vi "IOC shared memory de-initialize.vi"(0 "shared memory in":T2, 3 "Shared memory cluster":T1) -> ()   [LabVIEW 2020, in "linuxSharedMemory.lvlib"]
uses:
  linuxSharedMemory.lvlib
  <vilib>/NI/NI Linux RT IPC/Shared Memory/Controls/reference.ctl
  <vilib>/NI/NI Linux RT IPC/Shared Memory/Classes/Shared Memory/Shared Memory.lvclass
  controls/sm_cluster.ctl
  <vilib>/NI/NI Linux RT IPC/Shared Memory/Linux RT IPC.Shared Memory.lvlib
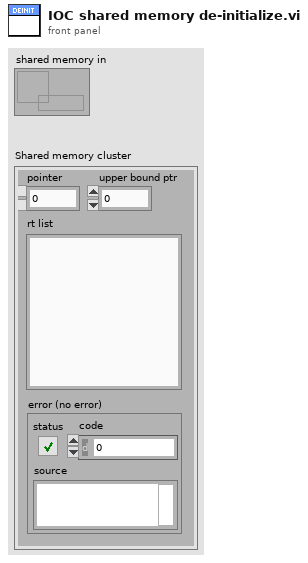
[diagram p1: front panel]
types:
  T1 = typedef "linuxSharedMemory.lvlib/sm_cluster.ctl" = cluster{"rt list":string, "error (no error)":errorcluster, "pointer":u64, "upper bound ptr":u64}
  T2 = typedef "Linux RT IPC.Shared Memory.lvlib/reference.ctl" = refnum<data-value>
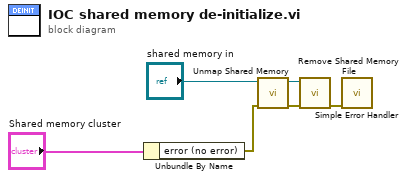
[diagram p0: block diagram]
diagram:
  n1 = Unbundle By Name("Shared memory cluster") -> ("error (no error)"=w1:errorcluster)
  n2 = call <vilib>:"Unmap Shared Memory.vi"("error in (no error)"=w1, "shared memory in"="shared memory in") -> ("error out"=w5:errorcluster, "shared memory out"=w4:T2)  [unwired: 8 in]
  n3 = call <vilib>:"Remove Shared Memory File.vi"("error in (no error)"=w5, "shared memory in"=w4) -> ("error out"=w6:errorcluster)  [unwired: 8 in, 1 out]
  n4 = call <vilib>:"Simple Error Handler.vi"("error in (no error)"=w6) -> ()  [unwired: 4 in, 5 out]
